vi "PathPlanner_Cmd_AutoInitFromJson.vi"(9 "Mirror":bool, 11 "JSON_String":string) -> (0 "error out":errorcluster, 3 "PathPlanner_Cmd_AutoConfig":T2 {"Paths"."IdealStartingState"."Rotation"."SIN" format="%13.4f"; "Paths"."IdealStartingState"."Rotation"."COS" format="%13.4f"; "Paths"."IdealStartingState"."Rotation"."VALUE" format="%13.4f"; "Paths"."PointTowardsZones"."TargetPosition"."Y" format="%14.3f"; "Paths"."PointTowardsZones"."TargetPosition"."X" format="%14.3f"; "Paths"."PointTowardsZones"."RotationOffset"."SIN" format="%13.4f"; "Paths"."PointTowardsZones"."RotationOffset"."COS" format="%13.4f"; "Paths"."PointTowardsZones"."RotationOffset"."VALUE" format="%13.4f"; "Paths"."Waypoints"."nextControl"."Y" format="%14.3f"; "Paths"."Waypoints"."nextControl"."X" format="%14.3f"; "Paths"."Waypoints"."anchor"."Y" format="%14.3f"; "Paths"."Waypoints"."anchor"."X" format="%14.3f"; "Paths"."Waypoints"."prevControl"."Y" format="%14.3f"; "Paths"."Waypoints"."prevControl"."X" format="%14.3f"; "Paths"."AllPoints"."RotationTarget"."rotation"."SIN" format="%13.4f"; "Paths"."AllPoints"."RotationTarget"."rotation"."COS" format="%13.4f"; "Paths"."AllPoints"."RotationTarget"."rotation"."VALUE" format="%13.4f"; "Paths"."AllPoints"."Position"."Y" format="%14.3f"; "Paths"."AllPoints"."Position"."X" format="%14.3f"; "Paths"."GoalEndState"."Rotation"."SIN" format="%13.4f"; "Paths"."GoalEndState"."Rotation"."COS" format="%13.4f"; "Paths"."GoalEndState"."Rotation"."VALUE" format="%13.4f"; "Paths"."RotationTargets"."rotation"."SIN" format="%13.4f"; "Paths"."RotationTargets"."rotation"."COS" format="%13.4f"; "Paths"."RotationTargets"."rotation"."VALUE" format="%13.4f"}, 4 "version":string)   [LabVIEW 2019, in "PathPlanner24.lvlib"]
doc: "DOCUMENTATION IS NOT COMPLETE.\n \nPack controller tuning configuration for Path Planner Holonomic Drive Controller.\n\nInputs:\n - X PID Tuning - cluster - Input from PACK PROF PID VI\n - Y PID Tuning - cluster - Input from PACK PROF PID VI\n - thetaController - cluster - A profiled PID controller to respond to error in angle.\n - Max Wheel Speed M/.S - double - Maximum wheel speed (M/S)\n - DriveBaseRadius - double - The radius of the drive base in meters. For swerve drive, this is the\n distance from the center of the robot to the furthest module. For \n mecanum, this is the drive base width / 2\n - X Tolerance - double - X tolerance for calculating At Reference (Meters) (Optional. Default: 0.0762 )\n - Y Tolerance - double - Y tolerance for calculating At Reference (Meters) (Optional. Default: 0.0762 )\n - Rotation Tolerance - double - Rotation tolerance for calculating At Reference (Degrees) (Optional. Default: 0.0)873)\n\nOutputs:\n -- PathPlannerHolCtrlConfig -- cluster - packed controller configuration."
uses:
  PathPlanner24.lvlib
  TypeDef/PathPlannerCmdPathPlannerAutoConfig.ctl
  TypeDef/PathPlannerCommandUtil.ctl
  ENum/PathPlanner_CommandUtil_Type_ENUM.ctl
  TypeDef/PathPlannerPath.ctl
  TypeDef/PathPlannerRotationTarget.ctl
  <vilib>/Rock Robotics/WPI/ThirdParty/JAS_Junk/TrajLib/TypeDef/ROTATION2D.ctl
  TypeDef/PathPlannerConstraintsZone.ctl
  TypeDef/PathPlannerPathConstraints.ctl
  TypeDef/PathPlannerEventMarker.ctl
  TypeDef/PathPlannerGoalEndState.ctl
  TypeDef/PathPlannerPathPoint.ctl
  <vilib>/Rock Robotics/WPI/ThirdParty/JAS_Junk/TrajLib/TypeDef/TRANSLATION2D.ctl
  TypeDef/PathPlannerWaypoint.ctl
  TypeDef/PathPlannerPointTowardsZone.ctl
  TypeDef/PathPlannerIdealStartingState.ctl
  PathPlanner_IdealStartingState_New.vi
  <vilib>/Rock Robotics/WPI/ThirdParty/JAS_Junk/TrajLib/Rotation2d_UnaryMinus.vi
  PathPlanner_IdealStartingState_GetAll.vi
  PathPlanner_Path_MirrorTranslation.vi
  PathPlanner_RotationTarget_GetAll.vi
  PathPlanner_RotationTarget_New.vi
  PathPlanner_PointTowardsZone_New.vi
  PathPlanner_GoalEndState_GetAll.vi
  PathPlanner_GoalEndState_New.vi
  PathPlanner_PathPoint_GetAll.vi
  PathPlanner_PathPoint_New.vi
  PathPlanner_PathPoint_SetWaypointRelPos.vi
  <vilib>/Rock Robotics/WPI/ThirdParty/JAS_Junk/TrajLib/Rotation2d_CreateAngle.vi
  <vilib>/Rock Robotics/WPI/ThirdParty/JAS_Junk/TrajLib/Translation2d_GetXY.vi
  <vilib>/Rock Robotics/WPI/ThirdParty/JAS_Junk/TrajLib/Translation2d_Create.vi
  PathPlanner_FieldUtil_FieldSizeY.vi
  <vilib>/Rock Robotics/WPI/ThirdParty/JAS_Junk/TrajLib/Conv_Feet_Meters.vi
  PathPlanner_Path_FromPathFile.vi
  <vilib>/Rock Robotics/WPI/ThirdParty/JAS_Junk/TrajLib/Trajectory_Library.lvlib
panel:
  in  "?":T1
  out "Exists":bool
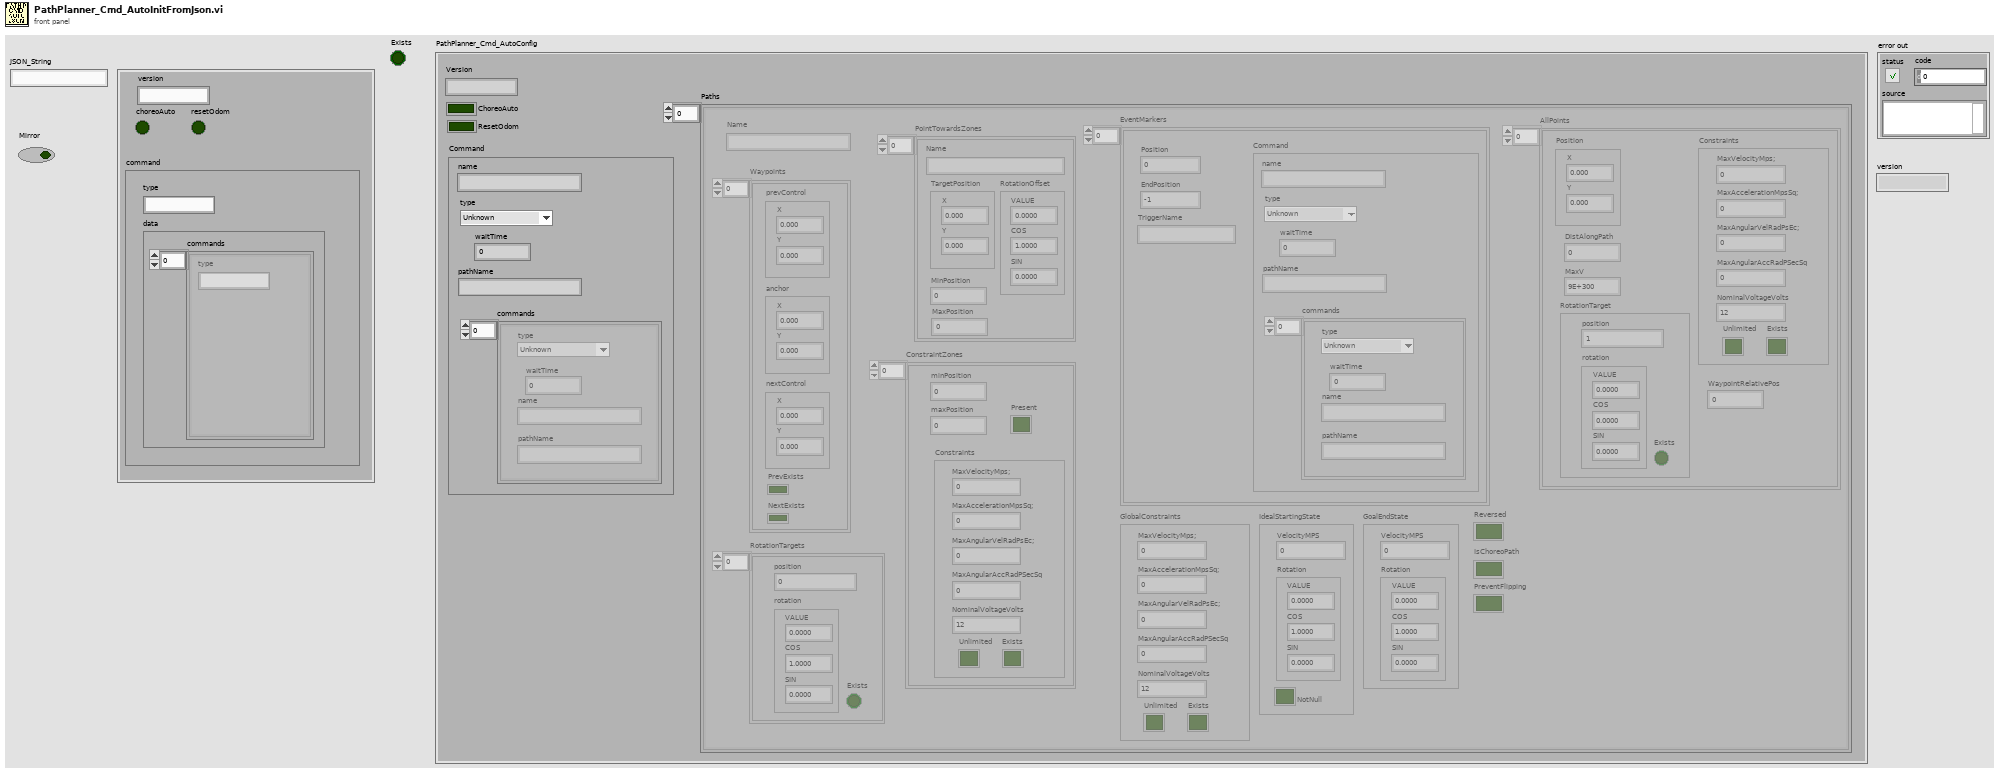
[diagram p1: front panel]
types:
  T1 = cluster{"version":string, "command":cluster{"type":string, "data":cluster{"commands":cluster{"type":string}[]}}, "resetOdom":bool, "choreoAuto":bool}
  T2 = typedef "PathPlanner24.lvlib/PathPlannerCmdPathPlannerAutoConfig.ctl" = cluster{"Command":T3, "ChoreoAuto":bool, "Version":string, "ResetOdom":bool, "Paths":T5[]}
  T3 = typedef "PathPlanner24.lvlib/PathPlannerCommandUtil.ctl" = cluster{"waitTime":dbl, "name":string, "pathName":string, "commands":cluster{"type":T4, "waitTime":dbl, "name":string, "pathName":string}[], "type":T4}
  T4 = typedef "PathPlanner24.lvlib/PathPlanner_CommandUtil_Type_ENUM.ctl" = enum16{"Unknown", "Wait", "Named", "Path", "Sequential", "Parallel", "Race", "Deadline", "PointTowardsZoneEnter", "PointTowardsZoneExit", "TriggerEventStart", "TriggerEventStop", "TriggerEventOneshot"}
  T5 = typedef "PathPlanner24.lvlib/PathPlannerPath.ctl" = cluster{"Reversed":bool, "RotationTargets":T6[], "ConstraintZones":T8[], "EventMarkers":T10[], "GlobalConstraints":T9, "GoalEndState":T11, "AllPoints":T12[], "Name":string, "Waypoints":T14[], "PointTowardsZones":T15[], "IdealStartingState":T16, "IsChoreoPath":bool, "PreventFlipping":bool}
  T6 = typedef "PathPlanner24.lvlib/PathPlannerRotationTarget.ctl" = cluster{"position":dbl, "rotation":T7, "Exists":bool}
  T7 = typedef "Trajectory_Library.lvlib/ROTATION2D.ctl" = cluster{"VALUE":dbl, "COS":dbl, "SIN":dbl}
  T8 = typedef "PathPlanner24.lvlib/PathPlannerConstraintsZone.ctl" = cluster{"minPosition":dbl, "maxPosition":dbl, "Constraints":T9, "Present":bool}
  T9 = typedef "PathPlanner24.lvlib/PathPlannerPathConstraints.ctl" = cluster{"MaxVelocityMps;":dbl, "MaxAccelerationMpsSq;":dbl, "MaxAngularVelRadPsEc;":dbl, "MaxAngularAccRadPSecSq":dbl, "Exists":bool, "Unlimited":bool, "NominalVoltageVolts":dbl}
  T10 = typedef "PathPlanner24.lvlib/PathPlannerEventMarker.ctl" = cluster{"Position":dbl, "Command":T3, "TriggerName":string, "EndPosition":dbl}
  T11 = typedef "PathPlanner24.lvlib/PathPlannerGoalEndState.ctl" = cluster{"VelocityMPS":dbl, "Rotation":T7}
  T12 = typedef "PathPlanner24.lvlib/PathPlannerPathPoint.ctl" = cluster{"Position":T13, "DistAlongPath":dbl, "MaxV":dbl, "Constraints":T9, "RotationTarget":T6, "WaypointRelativePos":dbl}
  T13 = typedef "Trajectory_Library.lvlib/TRANSLATION2D.ctl" = cluster{"X":dbl, "Y":dbl}
  T14 = typedef "PathPlanner24.lvlib/PathPlannerWaypoint.ctl" = cluster{"prevControl":T13, "anchor":T13, "nextControl":T13, "PrevExists":bool, "NextExists":bool}
  T15 = typedef "PathPlanner24.lvlib/PathPlannerPointTowardsZone.ctl" = cluster{"RotationOffset":T7, "Name":string, "TargetPosition":T13, "MinPosition":dbl, "MaxPosition":dbl}
  T16 = typedef "PathPlanner24.lvlib/PathPlannerIdealStartingState.ctl" = cluster{"VelocityMPS":dbl, "Rotation":T7, "NotNull":bool}
  T17 = cluster{"type":T4, "waitTime":dbl, "name":string, "pathName":string}[]
  T18 = cluster{"type":T4, "waitTime":dbl, "name":string, "pathName":string}
  T19 = cluster{"type":string, "data":cluster{"commands":cluster{"type":string}[]}}
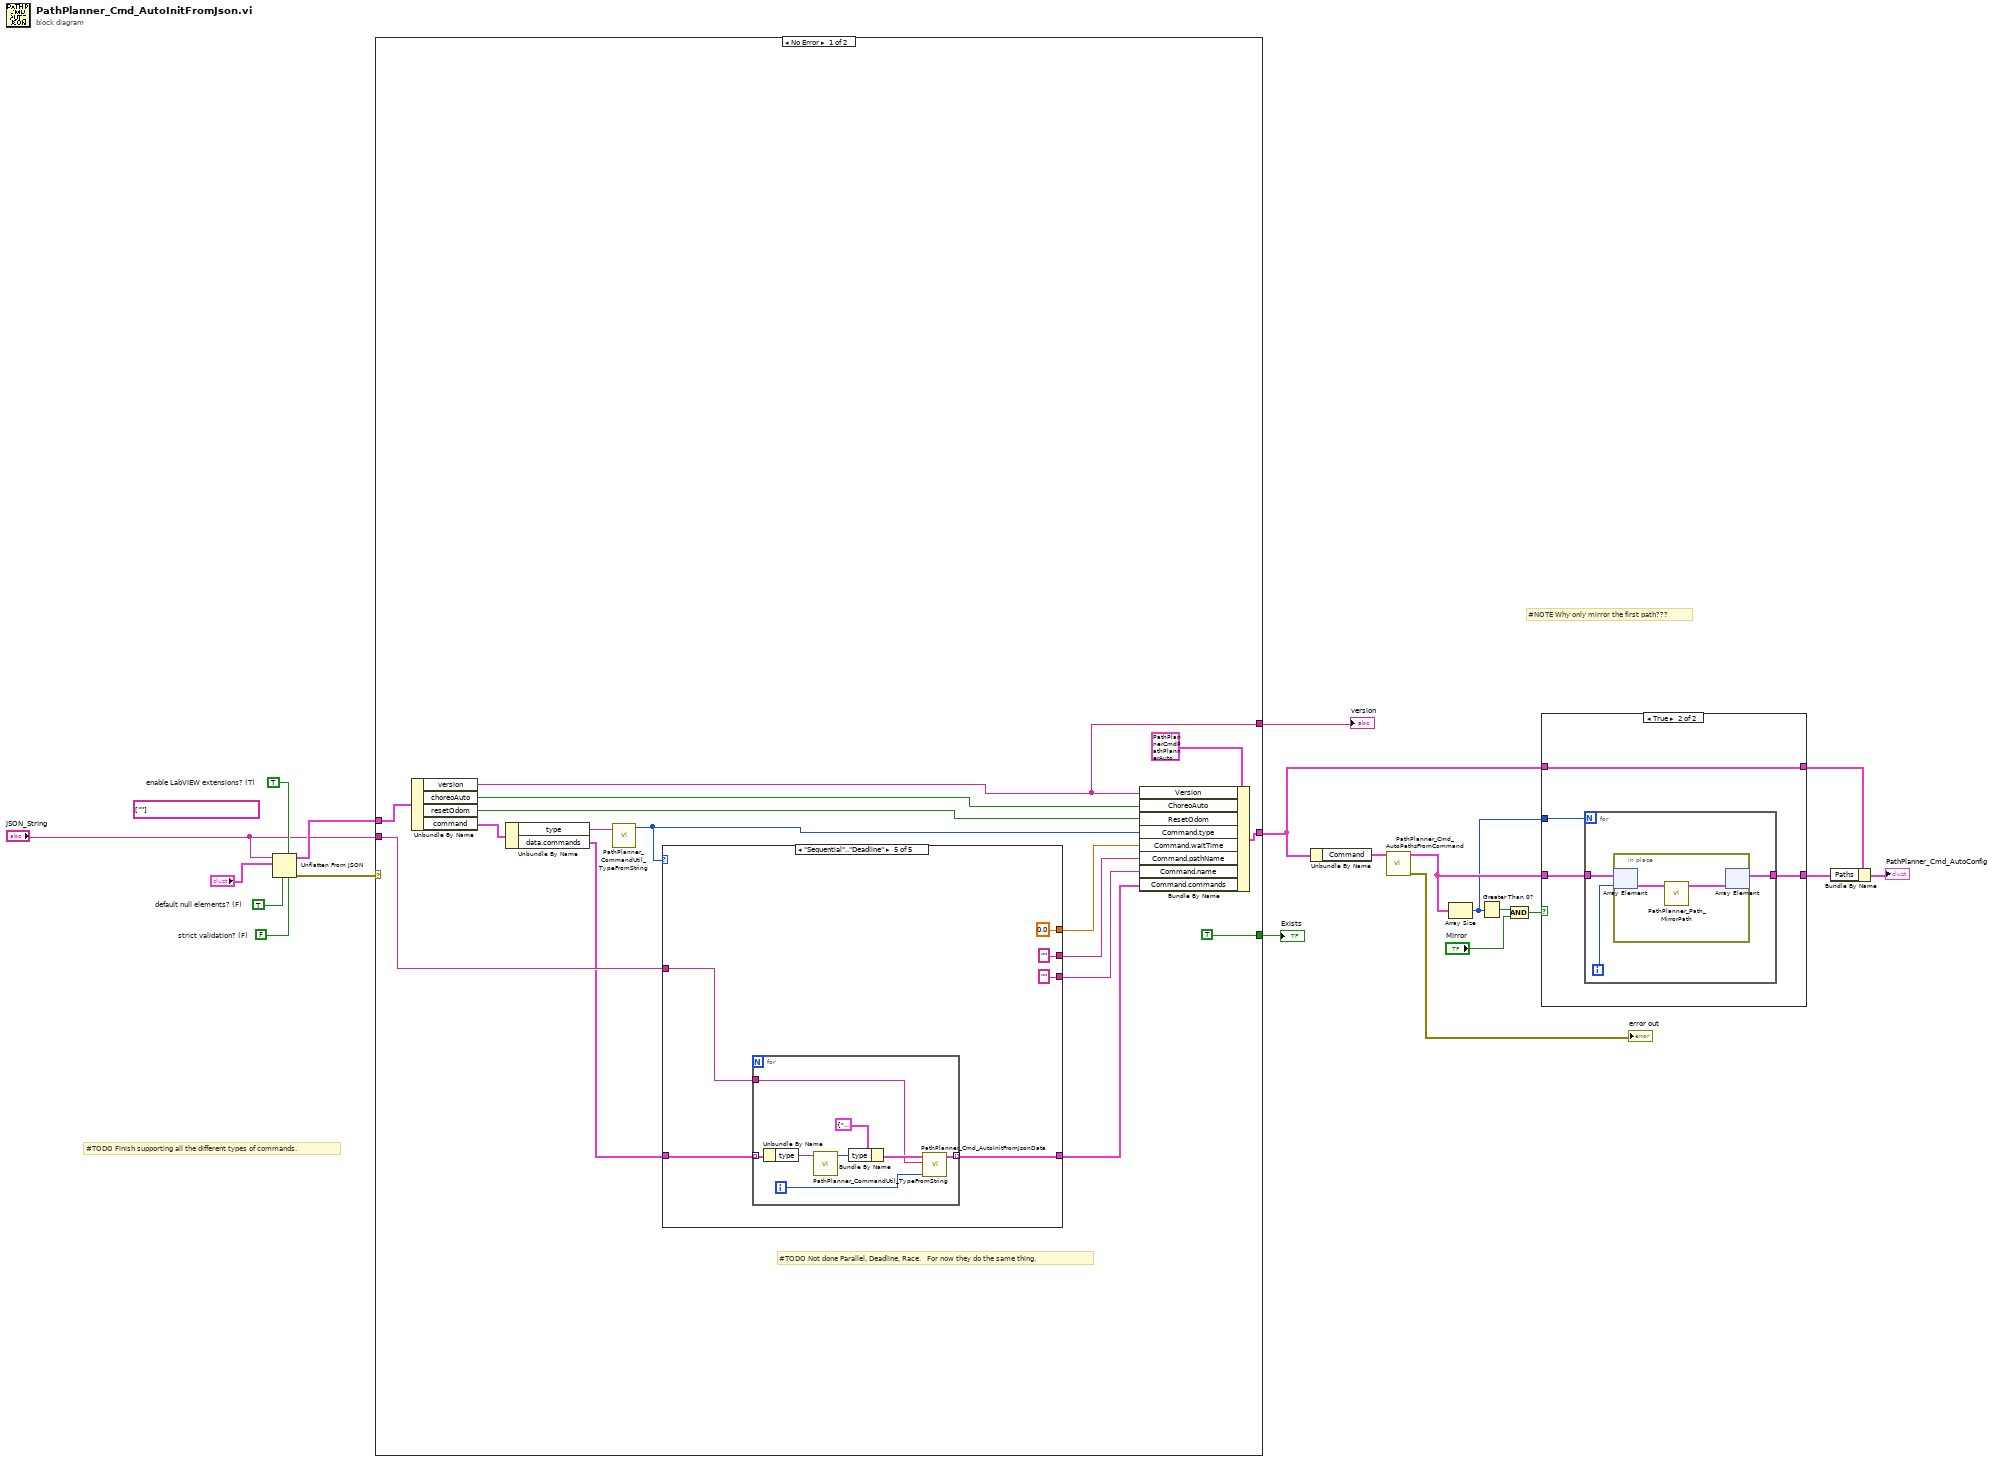
[diagram p0: block diagram]
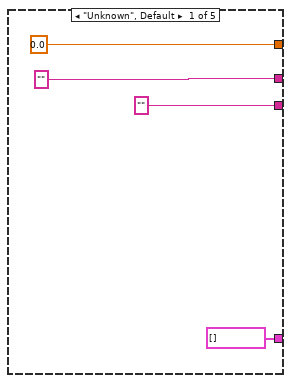
[diagram p3: hidden frame]
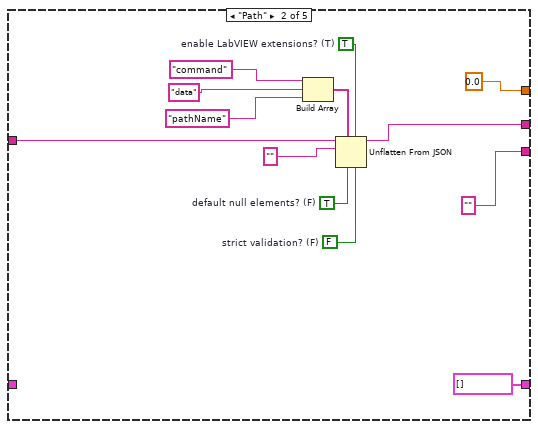
[diagram p4: hidden frame]
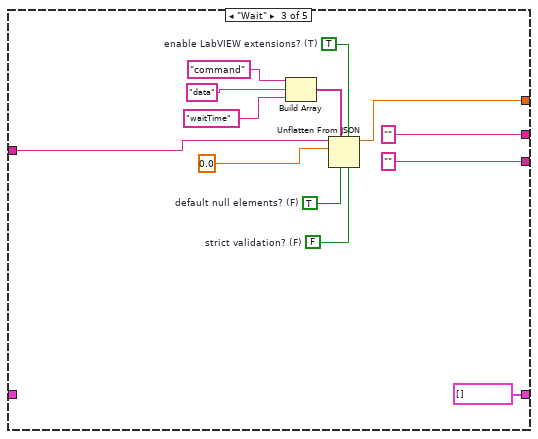
[diagram p5: hidden frame]
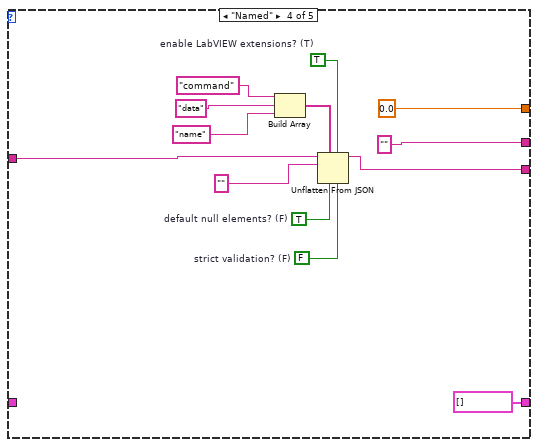
[diagram p6: hidden frame]
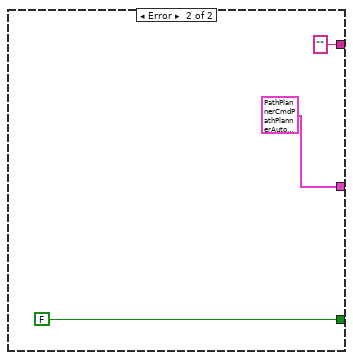
[diagram p7: hidden frame]
diagram:
  w18 = FALSE  # strict validation? (F)
  w19 = TRUE  # default null elements? (F)
  (unwired) string[] [""] ("path 2")
  w20 = TRUE  # enable LabVIEW extensions? (T)
  # "#NOTE Why only mirror the first path???"
  # "#TODO Finish supporting all the different types of commands."
  n1 = Unflatten From JSON(enable LabVIEW extensions? (T)=w20, JSON string="JSON_String", type and defaults="?", default null elements? (F)=w19, strict validation? (F)=w18) -> (value=w16:T1, error out=w17:errorcluster)  [unwired: 2 in]
  n2 = case shown="No Error" w17 {
    tunnel: w16 -> [w36 _]
    tunnel: [TRUE FALSE] -> w14
    tunnel: "JSON_String" -> [w29 _]
    tunnel: [w31 T2 {"Command"={"waitTime"=0.0, "name"="", "pathName"="", "commands"=[], "type"=enum."Unknown"}, "ChoreoAuto"=FALSE, "Version"="", "ResetOdom"=FALSE, "Paths"=[]} ("PathPlanner_Cmd_AutoConfig")] -> w3
    tunnel: [w26 "" ("version")] -> w9
    frame No Error {
      # "#TODO Not done Parallel, Deadline, Race.   For now they do the same thing."
      n3 = Unbundle By Name(w36) -> ("version"=w26:string, "choreoAuto"=w33:bool, "resetOdom"=w32:bool, "command"=w25:T19)
      n4 = Unbundle By Name(w25) -> ("type"=w24:string, "data.commands"=w22:cluster{"type":string}[])
      n5 = call "PathPlanner_CommandUtil_TypeFromString.vi"("Type string"=w24) -> ("Type"=w30:T4)  [unwired: 10 in]
      n6 = case shown="\"Sequential\"..\"Deadline\"" w30 {
        tunnel: w29 -> [_ w49 w59 w72 w84]
        tunnel: ["" w44 "" "" ""] -> w28
        tunnel: [0.0 0.0 w57 0.0 0.0] -> w27
        tunnel: ["" "" "" w68 ""] -> w23
        tunnel: w22 -> [_ _ _ _ w85]
        tunnel: [T17 [] T17 [] T17 [] T17 [] w83] -> w21
        frame "Unknown", Default {
        }
        frame "Path" {
          w51 = FALSE  # strict validation? (F)
          w52 = TRUE  # default null elements? (F)
          w53 = TRUE  # enable LabVIEW extensions? (T)
          n7 = Build Array("command", "data", "pathName") -> (w48:string[])
          n8 = Unflatten From JSON(path=w48, enable LabVIEW extensions? (T)=w53, JSON string=w49, type and defaults="", default null elements? (F)=w52, strict validation? (F)=w51) -> (value=w44:string)  [unwired: 1 in, 1 out]
        }
        frame "Wait" {
          w64 = FALSE  # strict validation? (F)
          w65 = TRUE  # default null elements? (F)
          w66 = TRUE  # enable LabVIEW extensions? (T)
          n9 = Build Array("command", "data", "waitTime") -> (w63:string[])
          n10 = Unflatten From JSON(path=w63, enable LabVIEW extensions? (T)=w66, JSON string=w59, type and defaults=0.0, default null elements? (F)=w65, strict validation? (F)=w64) -> (value=w57:dbl)  [unwired: 1 in, 1 out]
        }
        frame "Named" {
          w77 = FALSE  # strict validation? (F)
          w78 = TRUE  # default null elements? (F)
          w79 = TRUE  # enable LabVIEW extensions? (T)
          n11 = Build Array("command", "data", "name") -> (w76:string[])
          n12 = Unflatten From JSON(path=w76, enable LabVIEW extensions? (T)=w79, JSON string=w72, type and defaults="", default null elements? (F)=w78, strict validation? (F)=w77) -> (value=w68:string)  [unwired: 1 in, 1 out]
        }
        frame "Sequential".."Deadline" {
          n13 = for {
            tunnel: w85 -> [w93] mode=indexing
            tunnel: [w88] -> w83 mode=indexing
            tunnel: w84 -> [w87]
            i -> [w86]
            n14 = Unbundle By Name(w93) -> ("type"=w91:string)
            n15 = call "PathPlanner_CommandUtil_TypeFromString.vi"("Type string"=w91) -> ("Type"=w92:T4)  [unwired: 10 in]
            n16 = Bundle By Name(cluster=T18 {"type"=enum."Unknown", "waitTime"=0.0, "name"="", "pathName"=""} ("Command"), "type"=w92) -> (w89:T18)
            n17 = call "PathPlanner_Cmd_AutoInitFromJsonData.vi"("Cmd Index"=w86, "JSON String"=w87, "In Command Data"=w89) -> ("out Command Data"=w88:T18)  [unwired: 7 in, 1 out]
          }
        }
      }
      n18 = Bundle By Name(cluster=T2 {"Command"={"waitTime"=0.0, "name"="", "pathName"="", "commands"=[], "type"=enum."Unknown"}, "ChoreoAuto"=FALSE, "Version"="", "ResetOdom"=FALSE, "Paths"=[]} ("PathPlanner_Cmd_AutoConfig"), "Version"=w26, "ChoreoAuto"=w33, "ResetOdom"=w32, "Command.type"=w30, "Command.waitTime"=w27, "Command.pathName"=w28, "Command.name"=w23, "Command.commands"=w21) -> (w31:T2)
    }
    frame Error {
    }
  }
  "Exists" <- w14
  "version" <- w9
  n19 = Unbundle By Name(w3) -> ("Command"=w11:T3)
  n20 = call "PathPlanner_Cmd_AutoPathsFromCommand.vi"("CommandUtil"=w11) -> ("error out"=→"error out":errorcluster, "Paths"=w5:T5[])  [unwired: 9 in]
  n21 = Array Size(array=w5) -> (size(s)=w1:i32)
  n22 = Greater Than 0?(x=w1) -> (x > 0?=w8:bool)
  n23 = And(x=w8, y="Mirror") -> (x .and. y?=w6:bool)
  n24 = case shown="True" w6 {
    tunnel: w5 -> [w98 w100]
    tunnel: [w98 w102] -> w4
    tunnel: w3 -> [w97 w101]
    tunnel: [w97 w101] -> w2
    tunnel: w1 -> [_ w99]
    frame False {
    }
    frame True {
      n25 = for {
        N: w99 -> [_]
        tunnel: w100 -> [w105]
        tunnel: [w104] -> w102
        i -> [w103]
        n26 = in-place {
          n27 = in-place-array #1(w105, w103) -> (w107:T5)
          n28 = call "PathPlanner_Path_MirrorPath.vi"("in PathPlannerPath"=w107) -> ("out PathPlannerPath"=w106:T5)  [unwired: 10 in]
          n29 = in-place-array #1(w106) -> (w104:T5[])  [unwired: 1 out]
        }
      }
    }
  }
  n30 = Bundle By Name(cluster=w2, "Paths"=w4) -> (→"PathPlanner_Cmd_AutoConfig":T2)
